vi "DataReceiverphil5.vi"(4 "Acquisition Settings":T1, 5 "Network":T3={"invert_send"=TRUE, "Number of datagrams to read"=5000, "max bytes/read"=2500, "Timeout"=4000, "host"="192.168.1.18", "Port Receive"=5678} {"Number of datagrams to read" format="%0d"}, 6 "OK Button":bool) -> (0 "error out":errorcluster)   [LabVIEW 2014]
uses:
  testproj/controls/Network.ctl
  testproj/controls/DAQSettings.ctl
  testproj/controls/TriggerMode.ctl
panel:
  in  "error in":errorcluster
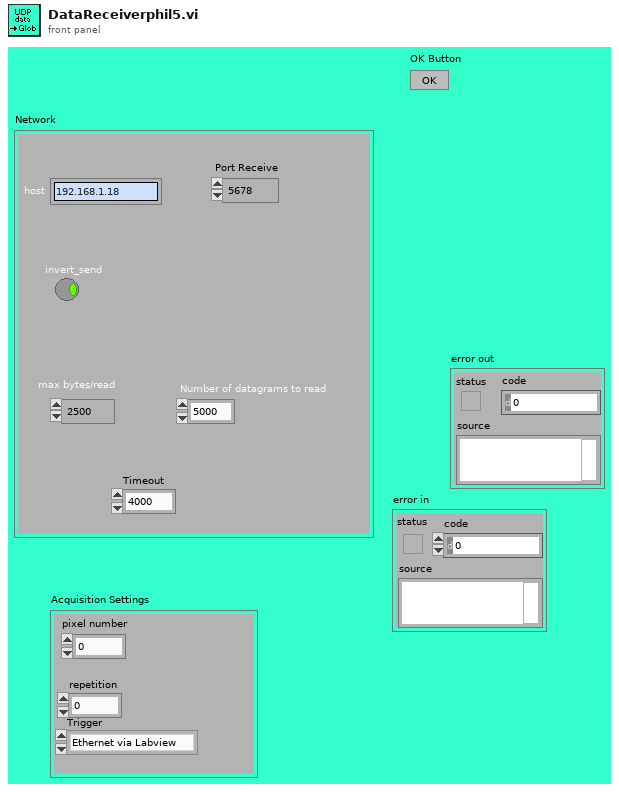
[diagram p1: front panel]
types:
  T1 = typedef "DAQSettings.ctl" = cluster{"pixel number":u32, "repetition":u32, "Trigger":T2}
  T2 = typedef "TriggerMode.ctl" = enum16{"Ethernet via Labview", "SMA (1.8V)"}
  T3 = typedef "Network.ctl" = cluster{"invert_send":bool, "Number of datagrams to read":u32, "max bytes/read":i32, "Timeout":i32, "host":string, "Port Receive":u16}
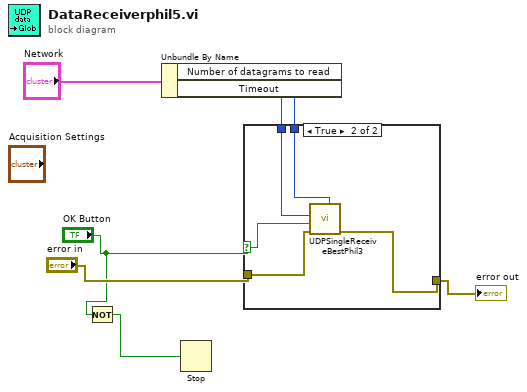
[diagram p0: block diagram]
diagram:
  n1 = Not(x="OK Button") -> (.not. x?=w1:bool)
  n2 = Unbundle By Name("Network") -> ("Number of datagrams to read"=w6:u32, "Timeout"=w5:i32)
  n3 = Stop(stop? (T)=w1) -> ()
  n4 = case shown="True" "OK Button" {
    selector: "OK Button" -> [_ w10]
    tunnel: [w8 w13] -> w4
    tunnel: w6 -> [_ w12]
    tunnel: w5 -> [_ w11]
    tunnel: "error in" -> [w8 w9]
    frame False {
    }
    frame True {
      n5 = call "UDPSingleReceiveBestPhil3.vi"("expectedRepetitions"=w12, "error in (no error)"=w9, "Boolean"=w10, "Timeout"=w11) -> ("error out"=w13:errorcluster)  [unwired: 4 in, 3 out]
    }
  }
  "error out" <- w4
